vi "Event.vi"() -> ()   [LabVIEW 2016]
panel:
  in  "stop":bool
  in  "Seek Forward Button":bool
  out "Boolean":bool
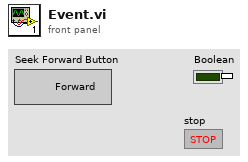
[diagram p1: front panel]
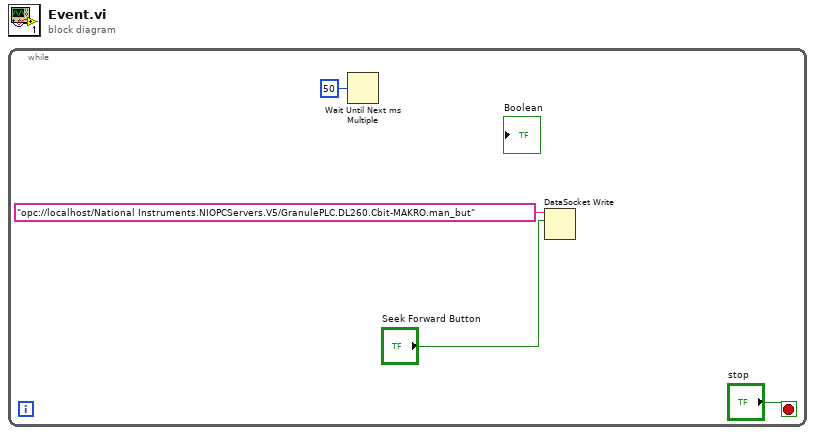
[diagram p0: block diagram]
diagram:
  n1 = while {
    stop <- "stop" stop-if-true
    n2 = Wait Until Next ms Multiple(millisecond multiple=u32 50) -> ()  [unwired: 1 out]
    n3 = DataSocket Write(10:"Seek Forward Button", 11:"opc://localhost/National Instruments.NIOPCServers.V5/GranulePLC.DL260.Cbit-MAKRO.man_but" ("connection in")) -> ()  [unwired: 2 in, 3 out]
  }
